vi "SVL Calibrate Microphone (DAQmx).vi"(0 "DAQmx physical channel":tag, 1 "calibration settings":T8={"calibration value [dB SPL]"=94.0, "calibration frequency [Hz]"=1000.0} {"calibration value [dB SPL]" format="%.2f"; "calibration frequency [Hz]" format="%.2f"}, 2 "channel configuration":T7={"maximum value (V)"=1.0, "minimum value (V)"=-1.0, "terminal configuration"=-1} {"terminal configuration" items=["Default"=-1, "RSE"=10083, "NRSE"=10078, "Differential"=10106, "Pseudodifferential"=12529]; "minimum value (V)" format="%.2f"; "maximum value (V)" format="%.2f"}, 3 "enable IEPE excitation (F)":bool, 4 "channel info":T9={"sensor sensitivity"=1000.0, "engineering units"=2, "dB reference"=2e-05, "custom label"="EU", "weighting filter"=0, "pregain"=0.0} {"pregain" format="%.2f"; "weighting filter" items=["Linear", "A-weighting", "B-weighting", "C-weighting", "ITU-R 468-4", "Dolby", "CCITT", "C-message", "Wb", "Wc", "Wd", "We", "Wf", "Wh", "Wj", "Wk", "Wm", "AES17 20 kHz lowpass", "AES17 40 kHz lowpass", "AES17 20 kHz highpass", "AES17 40 kHz highpass"]; "dB reference" format="%^.1e"; "engineering units" items=["custom..."=0, "V"=1, "A"=21, "C"=30, "pC"=31, "s"=32, "-"=29, "Pa"=2, "N"=20, "g"=3, "m/s^2"=4, "m/s"=5, "m"=6, "mm/s"=12, "mm"=13, "micron/s"=14, "micron"=15, "in/s^2"=7, "in/s"=8, "in"=9, "mil/s"=10, "mil"=11, "rad/s^2"=16, "rad/s"=17, "rad"=18, "deg/s^2"=26, "deg/s"=27, "deg"=28, "RPM"=22, "cycle/s^2"=23, "Hz"=24, "cycle"=25, "strain"=19]; "sensor sensitivity" format="%#_5f"}, 5 "error in (no error)":errorcluster, 6 "sampling frequency [Hz]":dbl=50000.0 format="%.2f", 7 "self calibrate device (F)":bool, 8 "duration [s]":dbl=1.0 format="%.2f", 9 "time to settle [s]":dbl format="%_2f", 11 "IEPE current [mA]":dbl=2.0 format="%_2f") -> (10 "power spectrum":cluster{"x0":dbl, "dx":dbl, "magnitude":dbl[]}(graph), 12 "spectrum info":T1={"channel name"="", "description"="", "x-axis units"=0, "spectral info"={"spectrum type"=enum."Power [Magnitude^2]", "linear/dB"=enum."linear", "window"=0, "window size"=0, "FFT size"=0}, "engineering units"=1, "custom label"="", "dB reference [EU]"=0.0, "peak units"=enum."rms", "weighting filter"=0, "spectral density?"=FALSE, "unit label"="", "spectrum skewed?"=FALSE, "complimentary spectrum units"=enum."none"} {"x-axis units" items=["Time (s)"=0, "Frequency-CB (Hz)"=1, "Frequency-CPB (Hz)"=1248, "Frequency-Arbitrary (Hz)"=2357, "Quefrency (s)"=2, "Revolutions (rev)"=3, "Order"=4, "Speed (RPM)"=11, "Speed (rad/s)"=21, "Index"=65535]; "weighting filter" items=["Linear", "A-weighting", "B-weighting", "C-weighting", "ITU-R 468-4", "Dolby", "CCITT", "C-message", "Wb", "Wc", "Wd", "We", "Wf", "Wh", "Wj", "Wk", "Wm", "AES17 20 kHz lowpass", "AES17 40 kHz lowpass", "AES17 20 kHz highpass", "AES17 40 kHz highpass"]; "dB reference [EU]" format="%.2f"; "engineering units" items=["custom..."=0, "V"=1, "A"=21, "C"=30, "pC"=31, "s"=32, "-"=29, "Pa"=2, "N"=20, "g"=3, "m/s^2"=4, "m/s"=5, "m"=6, "mm/s"=12, "mm"=13, "micron/s"=14, "micron"=15, "in/s^2"=7, "in/s"=8, "in"=9, "mil/s"=10, "mil"=11, "rad/s^2"=16, "rad/s"=17, "rad"=18, "deg/s^2"=26, "deg/s"=27, "deg"=28, "RPM"=22, "cycle/s^2"=23, "Hz"=24, "cycle"=25, "strain"=19]; "spectral info"."window" items=["None "=0, "Hanning"=1, "Hamming"=2, "Blackman-Harris"=3, "Exact Blackman"=4, "Blackman"=5, "Flat Top"=6, "4 Term B-Harris "=7, "7 Term B-Harris"=8, "Low Sidelobe"=9, "Force - Exponential"=10, "Gaussian"=62]}, 14 "calibrated sensor sensitivity [mV/Pa]":dbl=nan format="%.2g", 15 "calibrated channel info":T9={"sensor sensitivity"=nan, "engineering units"=2, "dB reference"=2e-05, "custom label"="EU", "weighting filter"=0, "pregain"=0.0} {"pregain" format="%.2f"; "weighting filter" items=["Linear", "A-weighting", "B-weighting", "C-weighting", "ITU-R 468-4", "Dolby", "CCITT", "C-message", "Wb", "Wc", "Wd", "We", "Wf", "Wh", "Wj", "Wk", "Wm", "AES17 20 kHz lowpass", "AES17 40 kHz lowpass", "AES17 20 kHz highpass", "AES17 40 kHz highpass"]; "dB reference" format="%^.1e"; "engineering units" items=["custom..."=0, "V"=1, "A"=21, "C"=30, "pC"=31, "s"=32, "-"=29, "Pa"=2, "N"=20, "g"=3, "m/s^2"=4, "m/s"=5, "m"=6, "mm/s"=12, "mm"=13, "micron/s"=14, "micron"=15, "in/s^2"=7, "in/s"=8, "in"=9, "mil/s"=10, "mil"=11, "rad/s^2"=16, "rad/s"=17, "rad"=18, "deg/s^2"=26, "deg/s"=27, "deg"=28, "RPM"=22, "cycle/s^2"=23, "Hz"=24, "cycle"=25, "strain"=19]; "sensor sensitivity" format="%#_5f"}, 16 "amplitude [V rms]":dbl=nan format="%.4f", 17 "frequency [Hz]":dbl=nan format="%.2f", 19 "error out":errorcluster)   [LabVIEW 2017, in "SoundVib_Calibration.lvlib"]
doc: "Performs an end-to-end calibration on the selected channel by measuring the actual sensitivity of the sensor connected to the channel and returns the measured sensor sensitivity."
uses:
  <vilib>/addons/Sound and Vibration/svt_Calibration/SoundVib_Calibration.lvlib
  <vilib>/addons/_NISVFA/_Shared subVIs/Controls/svc_Channel Info.ctl
  <vilib>/addons/_NISVFA/_Shared subVIs/Controls/svc_Engineering Units Text Ring.ctl
  <vilib>/addons/_NISVFA/_Shared subVIs/Controls/svc_Weighting Filter Text Ring.ctl
  <vilib>/addons/_NISVFA/_Shared subVIs/Controls/svc_Spectrum Info.ctl
  <vilib>/addons/_NISVFA/_Shared subVIs/Controls/svc_X-Axis Units.ctl
  <vilib>/addons/_NISVFA/_Shared subVIs/Controls/svc_Spectrum Type.ctl
  <vilib>/addons/_NISVFA/_Shared subVIs/Controls/svc_Complimentary Spectrum Units.ctl
  <vilib>/addons/_NISVFA/_Shared subVIs/Controls/svc_DSA Channel Settings.ctl
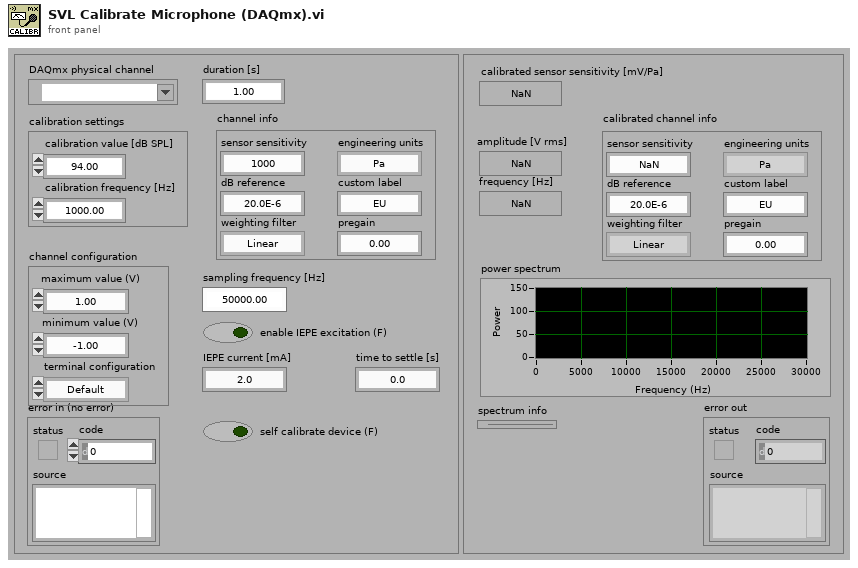
[diagram p1: front panel]
types:
  T1 = typedef "svc_Spectrum Info.ctl" = cluster{"channel name":string, "description":string, "x-axis units":T2, "spectral info":cluster{"spectrum type":T3, "linear/dB":enum16{"linear", "dB"}, "window":u16, "window size":i32, "FFT size":i32}, "engineering units":T4, "custom label":string, "dB reference [EU]":dbl, "peak units":enum16{"rms", "peak", "peak-peak"}, "weighting filter":T5, "spectral density?":bool, "unit label":string, "spectrum skewed?":bool, "complimentary spectrum units":T6}
  T2 = typedef "svc_X-Axis Units.ctl" = u16
  T3 = typedef "svc_Spectrum Type.ctl" = enum16{"FFT Spectrum [complex]", "Amplitude [Magnitude]", "Power [Magnitude^2]", "Cross Spectrum [complex]", "Frequency Response [Complex]"}
  T4 = typedef "svc_Engineering Units Text Ring.ctl" = u16
  T5 = typedef "svc_Weighting Filter Text Ring.ctl" = u16
  T6 = typedef "svc_Complimentary Spectrum Units.ctl" = enum16{"none", "radians", "degrees", "cycles", "imaginary"}
  T7 = cluster{"maximum value (V)":dbl, "minimum value (V)":dbl, "terminal configuration":i32}
  T8 = cluster{"calibration value [dB SPL]":dbl, "calibration frequency [Hz]":dbl}
  T9 = typedef "svc_Channel Info.ctl" = cluster{"sensor sensitivity":dbl, "engineering units":T4, "dB reference":dbl, "custom label":string, "weighting filter":T5, "pregain":dbl}
  T10 = typedef "svc_DSA Channel Settings.ctl" = cluster{"coupling":i32, "enable IEPE excitation":bool, "IEPE current [mA]":dbl}
  T11 = cluster{"calibration value [EUrms]":dbl, "calib. value is in dB (T)":bool, "calibration frequency [Hz]":dbl, "frequency tolerance [%]":dbl}
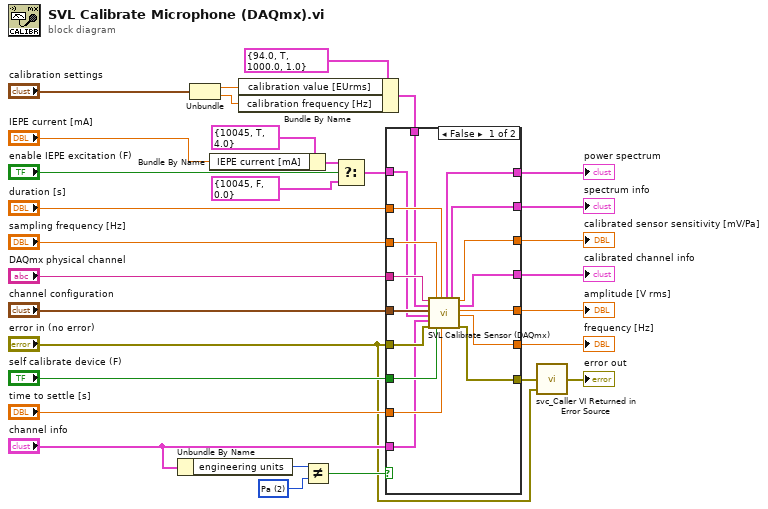
[diagram p0: block diagram]
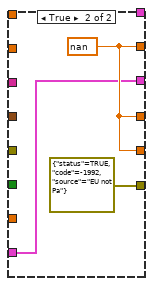
[diagram p2: hidden frame]
diagram:
  w13 = T4 2 items=["custom..."=0, "V"=1, "A"=21, "Pa"=2, "N"=20, "g"=3, "m/s^2"=4, "m/s"=5, "m"=6, "mm/s"=12, "mm"=13, "microns/s"=14, "microns"=15, "in/s^2"=7, "in/s"=8, "in"=9, "mils/s"=10, "mils"=11, "rad/s^2"=16, "rad/s"=17, "rad"=18, "strain"=19] ("y")
  n1 = Unbundle By Name("channel info") -> ("engineering units"=w14:T4)
  n2 = Unbundle("calibration settings") -> ("calibration value [dB SPL]"=w21:dbl, "calibration frequency [Hz]"=w16:dbl)
  n3 = Bundle By Name(cluster=T10 {"coupling"=10045, "enable IEPE excitation"=TRUE, "IEPE current [mA]"=4.0} ("DSA channel settings"), "IEPE current [mA]"="IEPE current [mA]") -> (w2:T10)
  n4 = Bundle By Name(cluster=T11 {"calibration value [EUrms]"=94.0, "calib. value is in dB (T)"=TRUE, "calibration frequency [Hz]"=1000.0, "frequency tolerance [%]"=1.0} ("calibration settings"), "calibration value [EUrms]"=w21, "calibration frequency [Hz]"=w16) -> (w24:T11)
  n5 = Not Equal?(x=w14, y=w13) -> (x != y?=w12:bool)
  n6 = Select(t=w2, s="enable IEPE excitation (F)", f=T10 {"coupling"=10045, "enable IEPE excitation"=FALSE, "IEPE current [mA]"=0.0} ("DSA channel settings")) -> (s? t:f=w6:T10)
  n7 = case shown="False" w12 {
    tunnel: "error in (no error)" -> [w47 _]
    tunnel: [w46 errorcluster {"status"=TRUE, "code"=-1992, "source"="EU not Pa"} ("error out")] -> w11
    tunnel: "self calibrate device (F)" -> [w45 _]
    tunnel: "time to settle [s]" -> [w44 _]
    tunnel: "DAQmx physical channel" -> [w43 _]
    tunnel: "sampling frequency [Hz]" -> [w42 _]
    tunnel: "duration [s]" -> [w41 _]
    tunnel: w24 -> [w40 _]
    tunnel: "channel configuration" -> [w39 _]
    tunnel: [w38 w50] -> w20
    tunnel: [w37 w49] -> w19
    tunnel: [w36 w50] -> w18
    tunnel: [w35 w50] -> w17
    tunnel: "channel info" -> [w34 w49]
    tunnel: w6 -> [w33 _]
    tunnel: [w32 _] -> w5
    tunnel: [w31 _] -> w4
    frame False {
      n8 = call <vilib>:"SVL Calibrate Sensor (DAQmx).vi"("DAQmx physical channel"=w43, "calibration settings"=w40, "channel configuration"=w39, "DSA channel settings"=w33, "channel info"=w34, "error in (no error)"=w47, "sampling frequency [Hz]"=w42, "self calibrate device (F)"=w45, "duration [s]"=w41, "time to settle [s]"=w44) -> ("power spectrum"=w32:cluster{"x0":dbl, "dx":dbl, "magnitude":dbl[]}, "spectrum info"=w31:T1, "calibrated sensor sensitivity [mV/EU]"=w38:dbl, "calibrated channel info"=w37:T9, "amplitude [V rms]"=w36:dbl, "frequency [Hz]"=w35:dbl, "error out"=w46:errorcluster)  [unwired: 3 in]
    }
    frame True {
      w50 = nan ("calibrated sensor sensitivity [mV/EU]")
    }
  }
  "amplitude [V rms]" <- w18
  "calibrated sensor sensitivity [mV/Pa]" <- w20
  "frequency [Hz]" <- w17
  "calibrated channel info" <- w19
  "power spectrum" <- w5
  "spectrum info" <- w4
  n9 = call <vilib>:"svc_Caller VI Returned in Error Source.vi"("warning input to caller"="error in (no error)", "error in (no error)"=w11) -> ("error out"=→"error out":errorcluster)  [unwired: 3 in]
